vi "Read Coords.vi"(8 "error in":errorcluster, 11 "XLS in":refnum<class "XLS.lvclass">=refnum) -> (0 "error out":errorcluster, 1 "Index":i32, 2 "Adr":string, 3 "XLS out":refnum<class "XLS.lvclass">)   [LabVIEW 2017, in "Reports.lvlib" / "XLS.lvclass"]
uses:
  XLS.lvclass
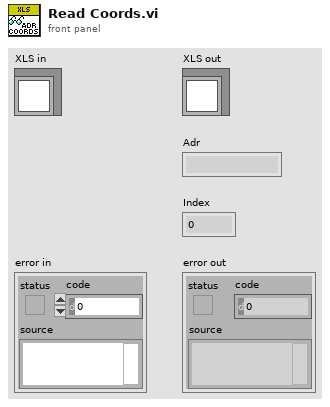
[diagram p1: front panel]
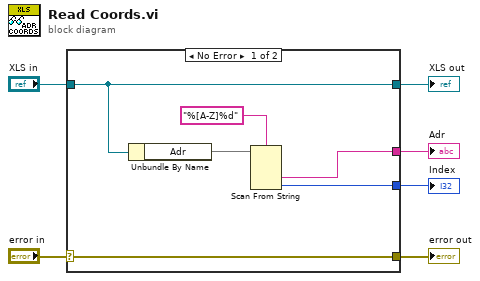
[diagram p0: block diagram]
diagram:
  n1 = case shown="No Error" "error in" {
    selector: "error in" -> [w12 w13]
    tunnel: [w12 w13] -> w5
    tunnel: [w11 w14] -> w3
    tunnel: "XLS in" -> [w11 w14]
    tunnel: [w8 _] -> w2
    tunnel: [w7 _] -> w1
    frame No Error {
      n2 = Unbundle By Name(w11) -> ("Adr"=w9)
      n3 = Scan From String(format string="%[A-Z]%d", input string=w9) -> (output 1=w8:string, output 2=w7:i32)  [unwired: 4 in, 3 out]
    }
    frame Error {
    }
  }
  "error out" <- w5
  "XLS out" <- w3
  "Index" <- w1
  "Adr" <- w2
